vi "Calc % Acquired.vi"(8 "error in (no error)":errorcluster, 11 "CCDCamera in":refnum<class "CCDCamera.lvclass">) -> (0 "error out":errorcluster, 3 "CCDCamera out":refnum<class "CCDCamera.lvclass">)   [LabVIEW 2018, in "CCDCamera.lvclass"]
uses:
  CCDCamera.lvclass
  CCDCamera.lvclass/CCDCamera.ctl
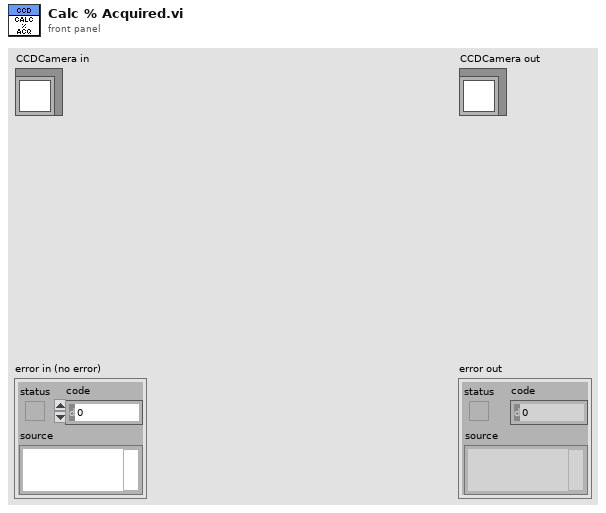
[diagram p1: front panel]
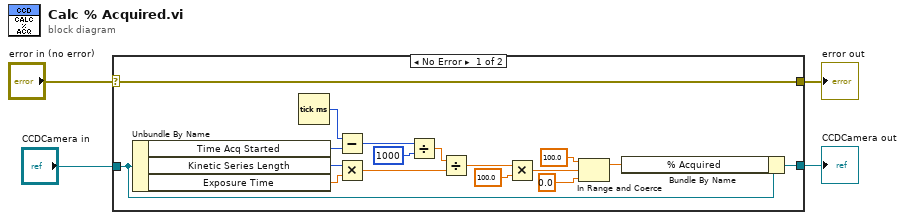
[diagram p0: block diagram]
diagram:
  n1 = case shown="No Error" "error in (no error)" {
    selector: "error in (no error)" -> [w21 w23]
    tunnel: [w21 w23] -> w3
    tunnel: [w15 w22] -> w1
    tunnel: "CCDCamera in" -> [w16 w22]
    frame No Error {
      n2 = Unbundle By Name(w16) -> ("Time Acq Started"=w19:u32, "Kinetic Series Length"=w7:u32, "Exposure Time"=w6:sgl)
      n3 = Tick Count (ms)() -> (millisecond timer value=w20:u32)
      n4 = Subtract(x=w20, y=w19) -> (x-y=w18:u32)
      n5 = Multiply(x=w7, y=w6) -> (x*y=w5:sgl)
      n6 = Divide(x=w18, y=1000) -> (x/y=w14:dbl)
      n7 = Divide(x=w14, y=w5) -> (x/y=w13:dbl)
      n8 = Multiply(x=w13, y=100.0) -> (x*y=w9:dbl)
      n9 = In Range and Coerce(upper limit=100.0, x=w9, lower limit=0.0) -> (coerced(x)=w8:dbl)  [unwired: 1 out]
      n10 = Bundle By Name(cluster=w16, "% Acquired"=w8) -> (w15:refnum<class "CCDCamera.lvclass">)
    }
    frame Error {
    }
  }
  "error out" <- w3
  "CCDCamera out" <- w1
